vi "List - Get First Selected Value.vi"(8 "Error In":errorcluster, 11 "List In":cluster{"Name":string, "Selected":bool}[](array[cluster])) -> (0 "Error Out":errorcluster, 2 "Index":i32, 3 "List Out":string[](array[string]))   [LabVIEW 2020]
doc: "This VI use to update selected value."
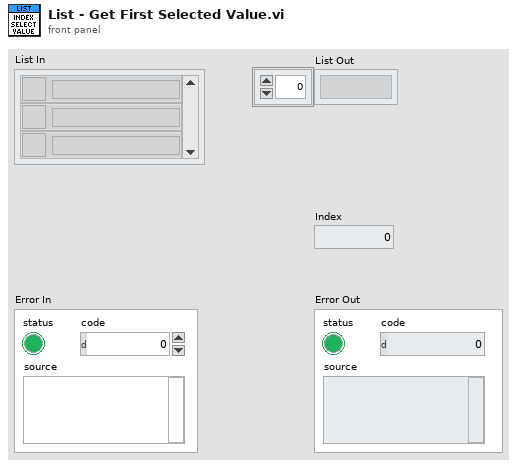
[diagram p1: front panel]
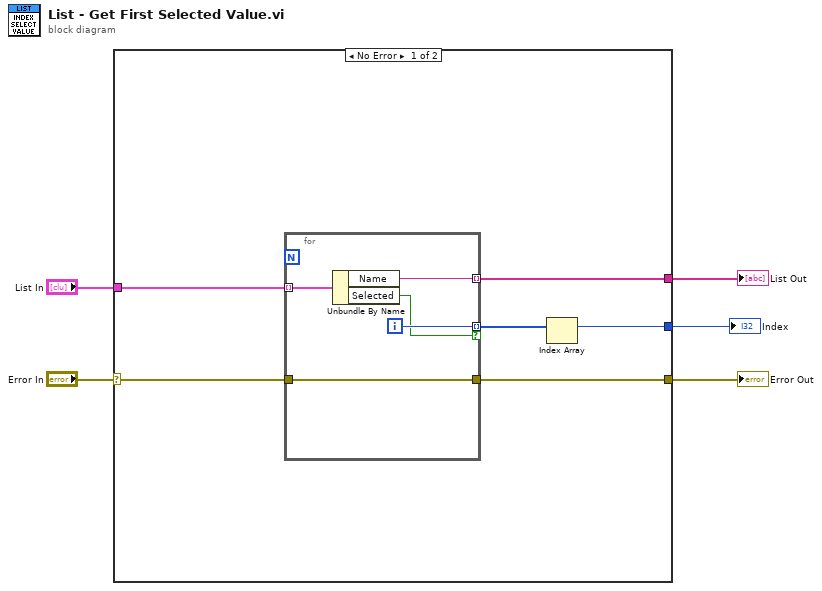
[diagram p0: block diagram]
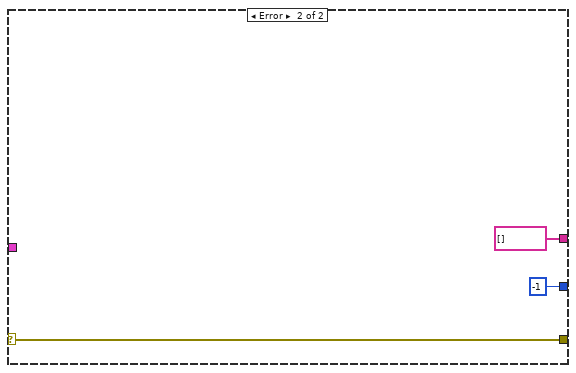
[diagram p2: hidden frame]
diagram:
  n1 = case shown="No Error" "Error In" {
    selector: "Error In" -> [w11 w19]
    tunnel: [w10 w19] -> w4
    tunnel: "List In" -> [w9 _]
    tunnel: [w8 string[] []] -> w2
    tunnel: [w6 -1] -> w1
    frame No Error {
      n2 = for {
        tunnel: w9 -> [w15] mode=indexing
        tunnel: [w16] -> w10
        tunnel: w11 -> [w16]
        tunnel: [w14] -> w8 mode=indexing
        tunnel: [w13] -> w7 mode=indexing if=w12
        i -> [w13]
        n3 = Unbundle By Name(w15) -> ("Name"=w14:string, "Selected"=w12:bool)
      }
      n4 = Index Array(array=w7) -> (element=w6:i32)  [unwired: 1 in]
    }
    frame Error {
    }
  }
  "Error Out" <- w4
  "List Out" <- w2
  "Index" <- w1
